vi "EjectMoney.vi"(8 "error in (no error)":errorcluster, 11 "object in":refnum<class "HasMoneyState.lvclass">) -> (0 "error out":errorcluster, 3 "object out":refnum<class "State.lvclass">)   [LabVIEW 2020, in "HasMoneyState.lvclass"]
uses:
  HasMoneyState.lvclass
  C:/Projects/DesignPatterns/StatePattern/State_class/State.lvclass
  State_class/State.lvclass
  <userlib>/_LabVIEWCommon/LcDialogs/LcDialog_AutoSizeDialog_Font.ctl
  NoMoneyState_class/NoMoneyState.lvclass
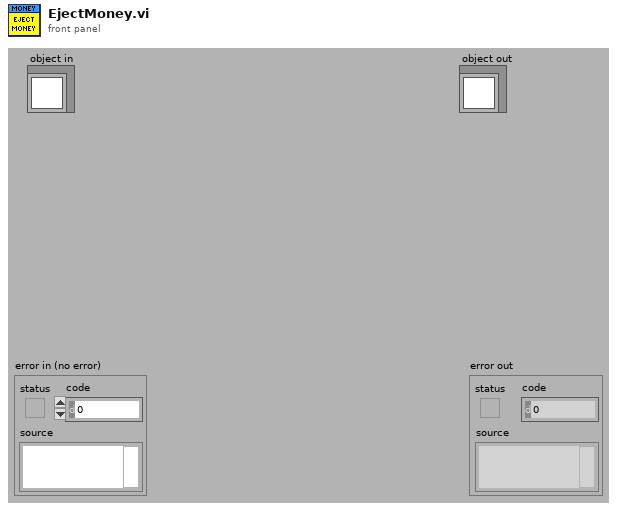
[diagram p1: front panel]
types:
  T1 = typedef "LcDialog_AutoSizeDialog_Font.ctl" = cluster{"Size":u32, "Bold":bool, "Color":u32}
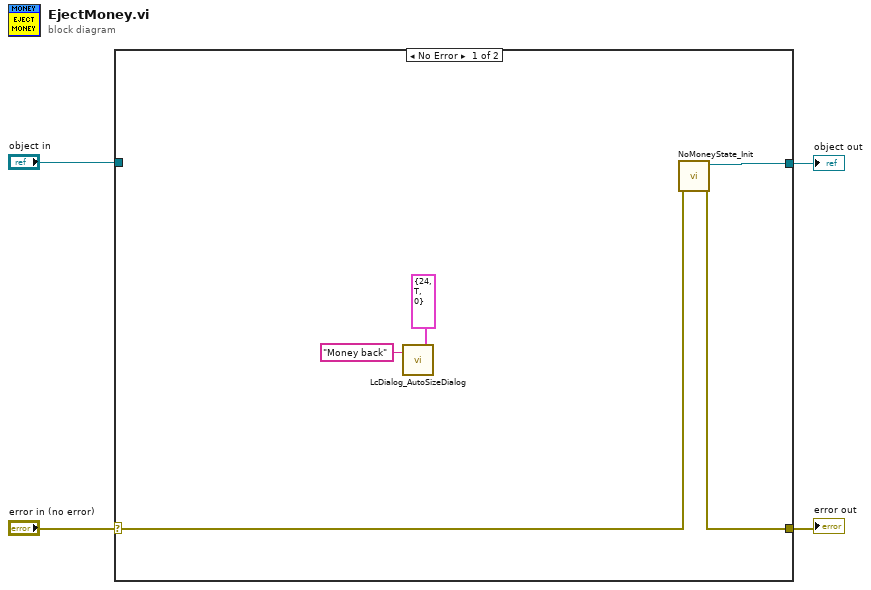
[diagram p0: block diagram]
diagram:
  n1 = case shown="No Error" "error in (no error)" {
    selector: "error in (no error)" -> [w8 w11]
    tunnel: [w7 w11] -> w3
    tunnel: [w9 w10] -> w1
    tunnel: "object in" -> [_ w10]
    frame No Error {
      n2 = call <userlib>:"LcDialog_AutoSizeDialog.vi"("TextIn"="Money back", "FontSettings"=T1 {"Size"=24, "Bold"=TRUE, "Color"=0}) -> ()  [unwired: 13 in, 5 out]
      n3 = call "NoMoneyState_Init.vi"("error in (no error)"=w8) -> ("error out"=w7:errorcluster, "object out"=w9:refnum<class "NoMoneyState.lvclass">)  [unwired: 9 in]
    }
    frame Error {
    }
  }
  "error out" <- w3
  "object out" <- w1
